vi "Remove_Spikes_Low.vi"(3 "index":i32, 4 "Background noise":dbl, 5 "Time Trace":dbl[](graph), 6 "Block Mean":dbl) -> (0 "Spike":bool, 1 "Filtered Time Trace":dbl[](graph), 2 "max value":dbl)   [LabVIEW 2018]
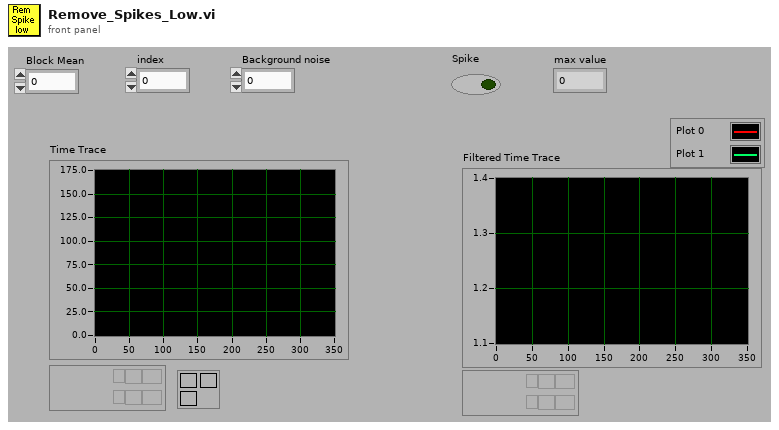
[diagram p1: front panel]
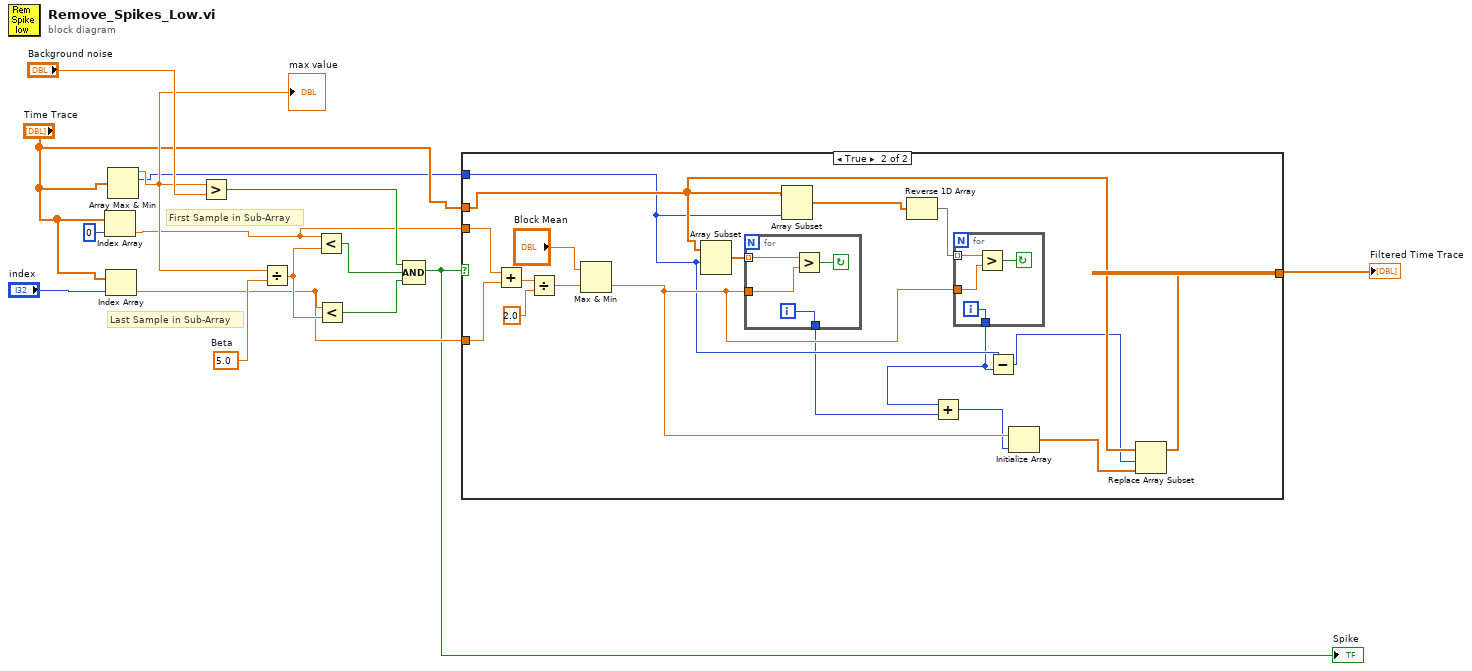
[diagram p0: block diagram]
diagram:
  w12 = 5.0  # Beta
  # "Last Sample in Sub-Array"
  # "First Sample in Sub-Array"
  n1 = Index Array(array="Time Trace", index=0) -> (element=w5:dbl)
  n2 = Index Array(array="Time Trace", index="index") -> (element=w4:dbl)
  n3 = Array Max & Min(array="Time Trace") -> (max value=w13:dbl, max index (indices)=w1:i32)  [unwired: 2 out]
  "max value" <- w13
  n4 = Greater?(x=w13, y="Background noise") -> (0:w10:bool)
  n5 = Divide(x=w13, y=w12) -> (x/y=w11:dbl)
  n6 = Less?(x=w5, y=w11) -> (x < y?=w9:bool)
  n7 = Less?(x=w4, y=w11) -> (x < y?=w8:bool)
  n8 = Compound Arithmetic op=AND(w10, w9, w8) -> (w3:bool)
  "Spike" <- w3
  n9 = case shown="True" w3 {
    tunnel: [w16 w25] -> w7
    tunnel: "Time Trace" -> [w16 w23]
    tunnel: w5 -> [_ w34]
    tunnel: w4 -> [_ w33]
    tunnel: w1 -> [_ w21]
    frame False {
    }
    frame True {
      n10 = Add(x=w34, y=w33) -> (x+y=w32:dbl)
      n11 = Divide(x=w32, y=2.0) -> (x/y=w29:dbl)
      n12 = Max & Min(x="Block Mean", y=w29) -> (min(x,y)=w27:dbl)  [unwired: 1 out]
      n13 = Array Subset(array=w23, index=w21) -> (w24:dbl[])  [unwired: 1 in]
      n14 = for {
        tunnel: w24 -> [w42] mode=indexing
        tunnel: w27 -> [w41]
        tunnel: [w39] -> w18
        i -> [w39]
        stop <- w40 continue-if-true
        n15 = Greater?(x=w42, y=w41) -> (0:w40:bool)
      }
      n16 = Array Subset(array=w23, length=w21) -> (w22:dbl[])  [unwired: 1 in]
      n17 = Reverse 1D Array(array=w22) -> (reversed array=w28:dbl[])
      n18 = for {
        tunnel: w28 -> [w38] mode=indexing
        tunnel: w27 -> [w37]
        tunnel: [w35] -> w19
        i -> [w35]
        stop <- w36 continue-if-true
        n19 = Greater?(x=w38, y=w37) -> (0:w36:bool)
      }
      n20 = Add(x=w19, y=w18) -> (x+y=w17:i32)
      n21 = Subtract(x=w21, y=w19) -> (x-y=w20:i32)
      n22 = Initialize Array(w27, w17) -> (w26:dbl[])
      n23 = Replace Array Subset(array=w23, new element=w26, index=w20) -> (w25:dbl[])
    }
  }
  "Filtered Time Trace" <- w7
